vi "WSVCAP SHL Host TL I2C Write - Multiple Device - Common Data.vi"(0 "Sub Address":u8=20 format="%.0x", 3 "FPGA":T1, 5 "Data Out [U8]":u8=20 format="%.0x", 11 "error in":errorcluster, 12 "Log (T)":bool=TRUE, 13 "DUT Mask Array (All)":bool[][](array[boolean])=[[TRUE, TRUE, TRUE, TRUE, TRUE, TRUE, TRUE, TRUE, TRUE, TRUE, TRUE, TRUE, TRUE, TRUE, TRUE, TRUE, TRUE, TRUE, TRUE, TRUE, TRUE, TRUE, TRUE, TRUE, TRUE, TRUE, TRUE, TRUE, TRUE, TRUE, TRUE, TRUE, TRUE, TRUE, TRUE, TRUE], [TRUE, TRUE, TRUE, TRUE, TRUE, TRUE, TRUE, TRUE, TRUE, TRUE, TRUE, TRUE, TRUE, TRUE, TRUE, TRUE, TRUE, TRUE, TRUE, TRUE, TRUE, TRUE, TRUE, TRUE, TRUE, TRUE, TRUE, TRUE, TRUE, TRUE, TRUE, TRUE, TRUE, TRUE, TRUE, TRUE], [TRUE, TRUE, TRUE, TRUE, TRUE, TRUE, TRUE, TRUE, TRUE, TRUE, TRUE, TRUE, TRUE, TRUE, TRUE, TRUE, TRUE, TRUE, TRUE, TRUE, TRUE, TRUE, TRUE, TRUE, TRUE, TRUE, TRUE, TRUE, TRUE, TRUE, TRUE, TRUE, TRUE, TRUE, TRUE, TRUE], [FALSE, FALSE, FALSE, FALSE, FALSE, FALSE, FALSE, FALSE, FALSE, FALSE, FALSE, FALSE, FALSE, FALSE, FALSE, FALSE, TRUE, FALSE, FALSE, FALSE, FALSE, FALSE, TRUE, FALSE, FALSE, FALSE, FALSE, FALSE, FALSE, FALSE, FALSE, TRUE, FALSE, FALSE, FALSE, FALSE]], 14 "DUT Mask Mode (All)":T2=enum."All") -> (15 "error out":errorcluster)   [LabVIEW 2012]
uses:
  Type Defs/WSVCAP SHL I2C DUT Mask Mode Enum.ctl
  Type Defs/WSVCAP SHL I2C FPGA Enum.ctl
panel:
  out "C3 Data Out":u8[](array[numeric]) format="%.0x"
  out "Socket Mask Set [U64]":u64[](array[numeric]) format="%012x"
  out "C2 Data Out":u8[](array[numeric]) format="%.0x"
  out "C1 Data Out":u8[](array[numeric]) format="%.0x"
  # "DUT 01"
  # "DUT 02"
  # "DUT 03"
  # "DUT 04"
  # "DUT 05"
  # "DUT 06"
  # "DUT 07"
  # "DUT 08"
  # "DUT 09"
  # "DUT 10"
  # "DUT 11"
  # "DUT 12"
  # "DUT 13"
  # "DUT 14"
  # "DUT 15"
  # "DUT 16"
  # "DUT 17"
  # "DUT 18"
  # "DUT 19"
  # "DUT 20"
  # "DUT 21"
  # "DUT 22"
  # "DUT 23"
  # "DUT 24"
  # "DUT 25"
  # "DUT 26"
  # "DUT 27"
  # "DUT 28"
  # "DUT 29"
  # "DUT 30"
  # "DUT 31"
  # "DUT 32"
  # "DUT 33"
  # "DUT 34"
  # "DUT 35"
  # "DUT 36"
  # "C1"
  # "C2"
  # "C3"
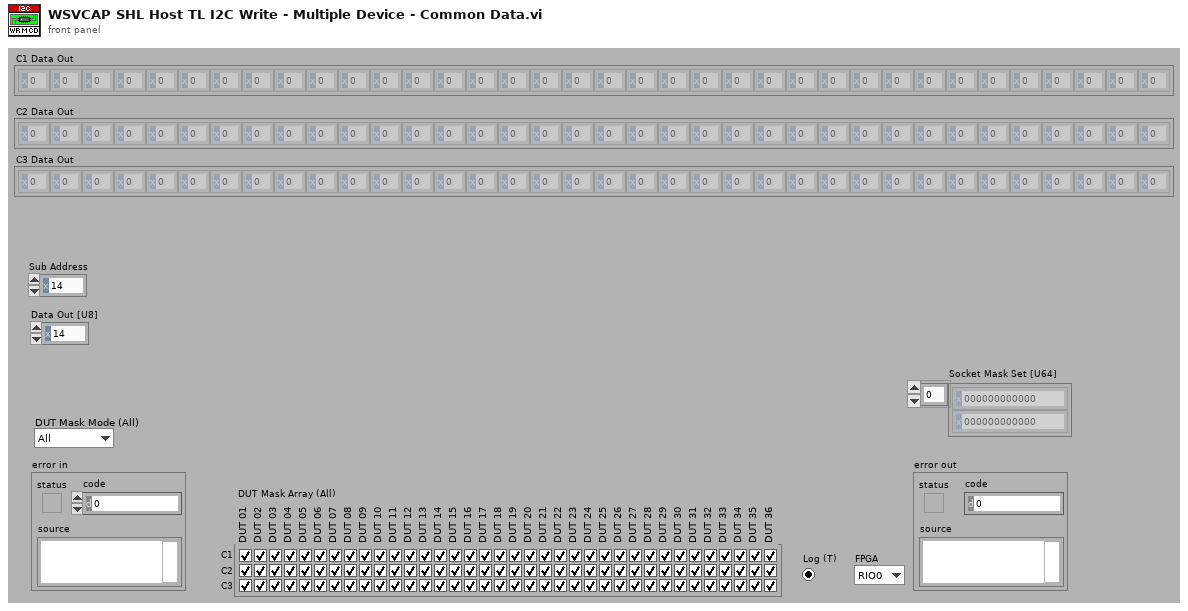
[diagram p1: front panel]
types:
  T1 = typedef "WSVCAP SHL I2C FPGA Enum.ctl" = enum16{"RIO0", "RIO1"}
  T2 = typedef "WSVCAP SHL I2C DUT Mask Mode Enum.ctl" = enum16{"Custom", "C1", "C2", "C3", "All"}
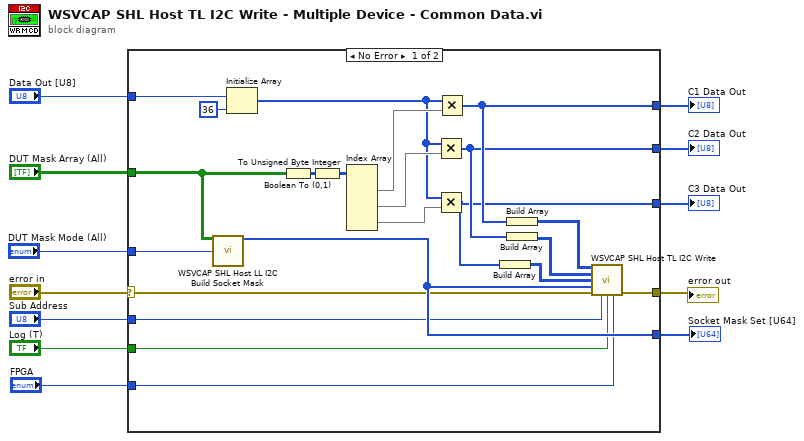
[diagram p0: block diagram]
diagram:
  n1 = case shown="No Error" "error in" {
    selector: "error in" -> [w22 w35]
    tunnel: [w34 w35] -> w12
    tunnel: "Sub Address" -> [w17 _]
    tunnel: "Data Out [U8]" -> [w29 _]
    tunnel: [w23 _] -> w8
    tunnel: [w24 _] -> w7
    tunnel: [w31 _] -> w6
    tunnel: "DUT Mask Array (All)" -> [w15 _]
    tunnel: "Log (T)" -> [w21 _]
    tunnel: [w16 _] -> w3
    tunnel: "DUT Mask Mode (All)" -> [w14 _]
    tunnel: "FPGA" -> [w13 _]
    frame No Error {
      n2 = call "WSVCAP SHL Host LL I2C Build Socket Mask.vi"("DUT Mask Array"=w15, "DUT Mask Mode (Custom)"=w14) -> ("Socket Mask Set [U64]"=w31:u64[])  [unwired: 13 in]
      n3 = Initialize Array(w29, 36 ("dimension size")) -> (w20:u8[])
      n4 = Boolean To (0,1)(Boolean=w15) -> (0, 1=w30:i16[][])
      n5 = To Unsigned Byte Integer(number=w30) -> (unsigned 8bit integer=w25:u8[][])
      n6 = Index Array(array=w25) -> (element #1=w27:u8[], element #2=w26:u8[], element #3=w19:u8[])  [unwired: 6 in]
      n7 = Multiply(x=w20, y=w26) -> (x*y=w23:u8[])
      n8 = Multiply(x=w20, y=w19) -> (x*y=w16:u8[])
      n9 = Multiply(x=w20, y=w27) -> (x*y=w24:u8[])
      n10 = Build Array(w16) -> (w18:u8[][])
      n11 = Build Array(w24) -> (w33:u8[][])
      n12 = Build Array(w23) -> (w32:u8[][])
      n13 = call "WSVCAP SHL Host TL I2C Write.vi"("C1 Data Out"=w33, "C2 Data Out"=w32, "C3 Data Out"=w18, "Socket Mask Set [U64]"=w31, "error in"=w22, "Sub Address"=w17, "Log (T)"=w21, "FPGA"=w13) -> ("error out"=w34:errorcluster)  [unwired: 7 in]
    }
    frame Error {
    }
  }
  "error out" <- w12
  "C1 Data Out" <- w7
  "C2 Data Out" <- w8
  "Socket Mask Set [U64]" <- w6
  "C3 Data Out" <- w3
